vi "HXG2-Error Handler - Main Handler.vi"(8 "error in (no error)":errorcluster, 11 "Message Queue":refnum<queue>) -> (3 "dup Message Queue":refnum<queue>)   [LabVIEW 2012]
uses:
  <userlib>/MessageQueue/Queue/Message Cluster.ctl
  <userlib>/MessageQueue/Queue/Message Queue.lvlib
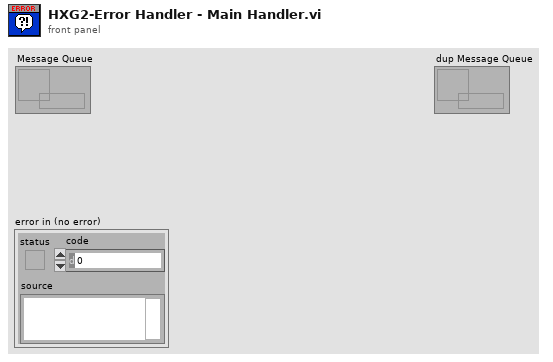
[diagram p1: front panel]
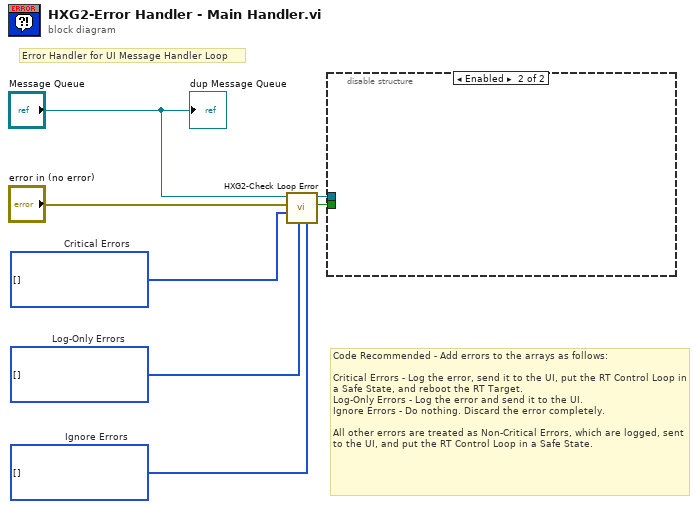
[diagram p0: block diagram]
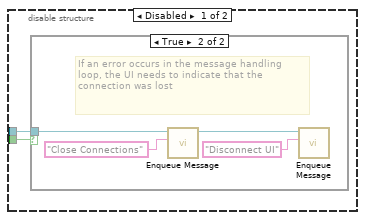
[diagram p2: hidden frame]
diagram:
  w3 = i32[] []  # Ignore Errors
  w4 = i32[] []  # Log-Only Errors
  w5 = i32[] []  # Critical Errors
  # "Code Recommended - Add errors to the arrays as follows:\n\nCritical Errors - Log the error, send it to the UI, put the RT Control Loop in a Safe State, and reboot the RT Target.\nLog-Only Errors - Log the error and send it to the UI.\nIgnore Errors - Do nothing. Discard the error completely.\n\nAll other errors are treated as Non-Critical Errors, which are logged, sent to the UI, and put the RT Control Loop in a Safe State."
  # "Error Handler for UI Message Handler Loop"
  n1 = call "HXG2-Check Loop Error.vi"("Ignore Errors"=w3, "Log-Only Errors"=w4, "Critical Errors"=w5, "error to process"="error in (no error)", "Message Queue"="Message Queue") -> ("Enqueued Error?"=w1:bool, "dup Message Queue"=w2:refnum<queue>)  [unwired: 5 in]
  n2 = disable-structure shown="Enabled" {
    disable-tunnel: w2 -> [w9 _]
    disable-tunnel: w1 -> [w8 _]
    frame Disabled {
      n3 = case shown="True" w8 {
        tunnel: w9 -> [_ w13]
        frame False {
        }
        frame True {
          # "If an error occurs in the message handling loop, the UI needs to indicate that the connection was lost"
          n4 = call <userlib>:"Enqueue Message.vi"("Message"="Close Connections", "Message Queue"=w13) -> ("dup Message Queue"=w11:refnum<queue>)  [unwired: 8 in, 1 out]
          n5 = call <userlib>:"Enqueue Message.vi"("Message"="Disconnect UI", "Message Queue"=w11) -> ()  [unwired: 8 in, 2 out]
        }
      }
    }
    frame Enabled {
    }
  }
  "dup Message Queue" <- "Message Queue"
